vi "Evaluate Uniform Cubic B-Spline.vi"(6 "starting index":i32, 9 "vertices v[0..m]":cdb[](array[numeric]), 10 "knots u[0..n]":dbl[](array[numeric]), 11 "u":dbl) -> (3 "curve value q[u]":cdb, 4 "knot index":i32)   [LabVIEW 2020, in "NI_Gmath.lvlib"]
uses:
  <vilib>/gmath/NI_Gmath.lvlib
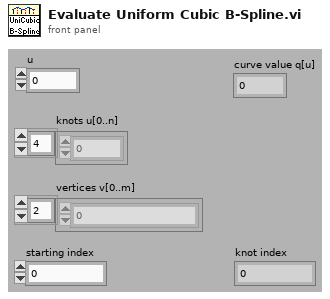
[diagram p1: front panel]
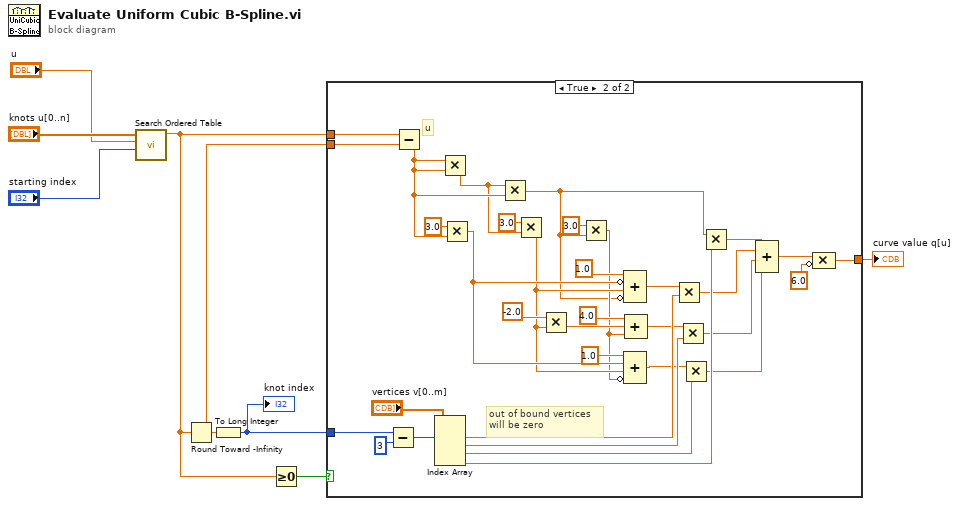
[diagram p0: block diagram]
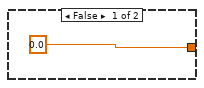
[diagram p2: hidden frame]
diagram:
  n1 = call <vilib>:"Search Ordered Table.vi"("starting index"="starting index", "x value"="u", "ordered x array"="knots u[0..n]") -> ("fractional index"=w2:dbl)  [unwired: 8 in]
  n2 = Round Toward -Infinity(1:w2) -> (0:w4:dbl)
  n3 = To Long Integer(number=w4) -> (32bit integer=w5:i32)
  "knot index" <- w5
  n4 = Greater Or Equal To 0?(x=w2) -> (x >= 0?=w3:bool)
  n5 = case shown="True" w3 {
    tunnel: w5 -> [_ w41]
    tunnel: w2 -> [_ w39]
    tunnel: w4 -> [_ w38]
    tunnel: [0.0 ("element") w10] -> w1
    frame False {
    }
    frame True {
      # "out of bound vertices\nwill be zero"
      # "u"
      n6 = Subtract(x=w41, y=3) -> (x-y=w42:i32)
      n7 = Subtract(x=w39, y=w38) -> (x-y=w36:dbl)
      n8 = Index Array(array="vertices v[0..m]", index #1=w42) -> (element #1=w23:cdb, element #2=w22:cdb, element #3=w19:cdb, element #4=w17:cdb)  [unwired: 3 in]
      n9 = Multiply(x=w36, y=w36) -> (x*y=w34:dbl)
      n10 = Multiply(x=3.0, y=w36) -> (x*y=w27:dbl)
      n11 = Multiply(x=w34, y=w36) -> (x*y=w18:dbl)
      n12 = Multiply(x=3.0, y=w34) -> (x*y=w26:dbl)
      n13 = Multiply(x=-2.0, y=w26) -> (x*y=w29:dbl)
      n14 = Multiply(x=3.0, y=w18) -> (x*y=w25:dbl)
      n15 = Compound Arithmetic op=ADD(1.0 ("x"), invert w27, w26, invert w18) -> (w24:dbl)
      n16 = Compound Arithmetic op=ADD(1.0 ("value"), w27, w26, invert w25) -> (w20:dbl)
      n17 = Compound Arithmetic op=ADD(4.0 ("x"), w29, w25) -> (w21:dbl)
      n18 = Multiply(x=w24, y=w23) -> (x*y=w15:cdb)
      n19 = Multiply(x=w21, y=w22) -> (x*y=w14:cdb)
      n20 = Multiply(x=w20, y=w19) -> (x*y=w13:cdb)
      n21 = Multiply(x=w18, y=w17) -> (x*y=w16:cdb)
      n22 = Compound Arithmetic op=ADD(w16, w15, w14, w13) -> (w11:cdb)
      n23 = Compound Arithmetic op=MULTIPLY(w11, invert 6.0 ("x")) -> (w10:cdb)
    }
  }
  "curve value q[u]" <- w1
